vi "Cuernitos Global.vi"() -> ()   [LabVIEW 2014]
panel:
  in  "Cuernitos":bool
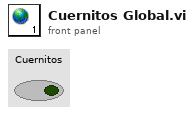
[diagram p1: front panel]
diagram:
